vi "Obtain Request Events.vi"(8 "error in":errorcluster, 10 "Create New? (F)":bool) -> (0 "error out":errorcluster, 2 "Sequence Engine Request Events":T1)   [LabVIEW 2021, in "Sequence Engine.lvlib"]
doc: "This VI Obtains/Creates the Requests events that will be used for other modules to communicate with the module that owns this VI. These Requests events will be accessed only via Public API methods for this module.\n\n<b>NOTE</b>: The contents of this VI are automatically generated and modified by the <b>Tools > DQMH Consortium > DQMH</b> utilities. Consider using those utilities instead of making your own modifications to this VI.\n_____\nBased on DQMH Dev Tools: Project Template 7.1.1.1528."
uses:
  Sequence Engine.lvlib
  Request Events--cluster.ctl
  Stop Argument--cluster.ctl
  Show Panel Argument--cluster.ctl
  Hide Panel Argument--cluster.ctl
  Get Module Execution Status Argument--cluster.ctl
  Show Diagram Argument--cluster.ctl
  REQ Run Sequence Argument--cluster.ctl
  Request to stop testing Argument--cluster.ctl
  Init Test Context Argument--cluster.ctl
  Sequence Context.ctl
  Classes/Sequence Engine/Sequence Engine.lvclass
panel:
  # "NOTE: The contents of this VI are automatically generated and modified by the Tools > DQMH Consortium > DQMH utilities. Consider using those utilities instead of making your own modifications to this VI."
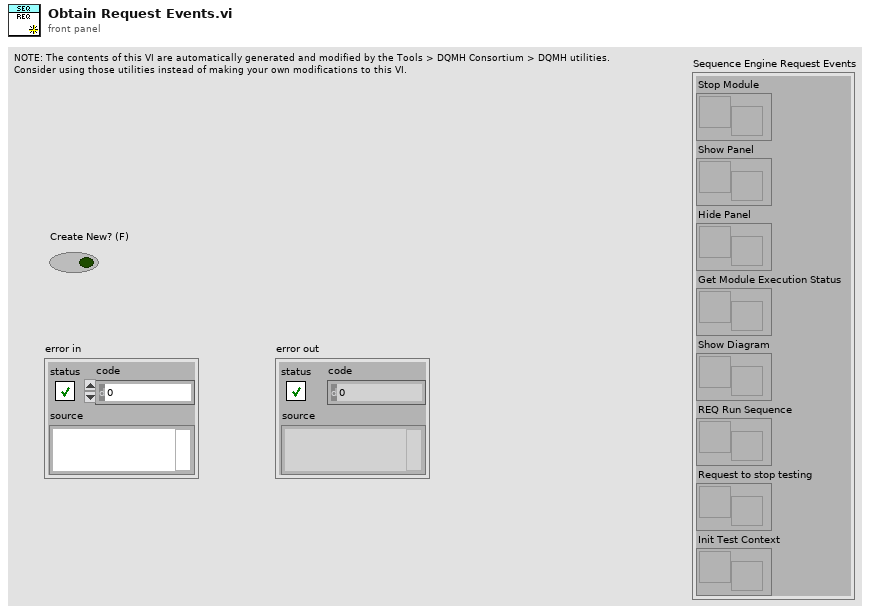
[diagram p1: front panel]
types:
  T1 = typedef "Sequence Engine.lvlib/Request Events--cluster.ctl" = cluster{"Stop Module":refnum<user-event>, "Show Panel":refnum<user-event>, "Hide Panel":refnum<user-event>, "Get Module Execution Status":refnum<user-event>, "Show Diagram":refnum<user-event>, "REQ Run Sequence":refnum<user-event>, "Request to stop testing":refnum<user-event>, "Init Test Context":refnum<user-event>}
  T2 = typedef "Sequence Engine.lvlib/Init Test Context Argument--cluster.ctl" = cluster{"Sequence Context":T3}
  T3 = typedef "Sequence Engine.lvlib/Sequence Engine.lvclass/Sequence Context.ctl" = cluster{"Execution Mode":enum16{"Production", "MSA1", "Trial"}, "Username":string, "Is Simulation":bool, "Hardware Map":string}
  T4 = typedef "Sequence Engine.lvlib/Request to stop testing Argument--cluster.ctl" = cluster{"Boolean":bool}
  T5 = typedef "Sequence Engine.lvlib/REQ Run Sequence Argument--cluster.ctl" = cluster{"Run.Start JSON":string}
  T6 = typedef "Sequence Engine.lvlib/Hide Panel Argument--cluster.ctl" = cluster{"Hide Panel?":bool}
  T7 = typedef "Sequence Engine.lvlib/Show Panel Argument--cluster.ctl" = cluster{"Show Panel?":bool}
  T8 = typedef "Sequence Engine.lvlib/Show Diagram Argument--cluster.ctl" = cluster{"Debug?":bool}
  T9 = typedef "Sequence Engine.lvlib/Get Module Execution Status Argument--cluster.ctl" = cluster{"Running?":bool}
  T10 = typedef "Sequence Engine.lvlib/Stop Argument--cluster.ctl" = cluster{"Origin":string, "Exit via Stop Module Req?":bool, "Wait for Module to stop?":bool}
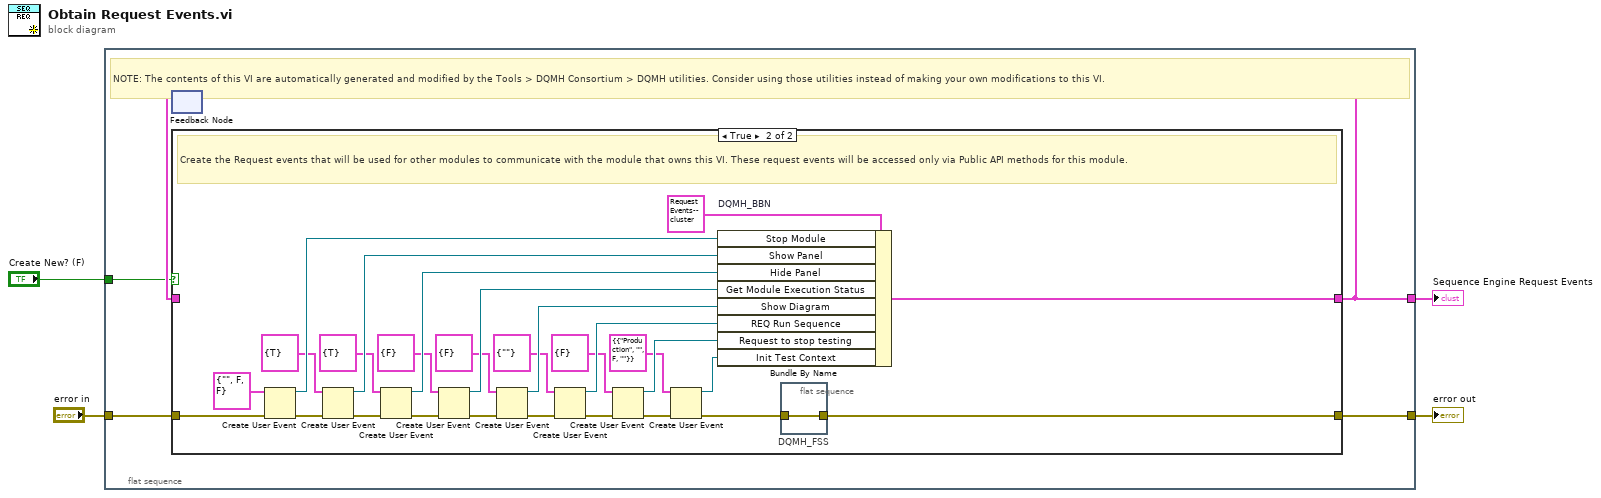
[diagram p0: block diagram]
diagram:
  n1 = flat-sequence {
    tunnel: [w9] -> w4
    tunnel: "error in" -> [w8]
    tunnel: [w6] -> w2
    tunnel: "Create New? (F)" -> [w5]
    frame #0 {
      # "NOTE: The contents of this VI are automatically generated and modified by the Tools > DQMH Consortium > DQMH utilities. Consider using those utilities instead of making your own modifications to this VI."
      n2 = feedback #1() -> (w7:T1)  [unwired: 1 in]
      n3 = case shown="True" w5 {
        tunnel: [w10 w29] -> w9
        tunnel: w8 -> [w10 w39]
        tunnel: [w11 w36] -> w6
        tunnel: w7 -> [w11 _]
        frame False {
          # "Obtain the Request events that were created in a previous call to this VI."
        }
        frame True {
          # "Create the Request events that will be used for other modules to communicate with the module that owns this VI. These request events will be accessed only via Public API methods for this module."
          n4 = Create User Event(user event datatype=T10 {"Origin"="", "Exit via Stop Module Req?"=FALSE, "Wait for Module to stop?"=FALSE} ("Stop Argument"), error in=w39) -> (user event=w37:refnum<user-event>, error out=w34:errorcluster)
          n5 = Create User Event(user event datatype=T7 {"Show Panel?"=TRUE} ("Show Panel Argument"), error in=w34) -> (user event=w33:refnum<user-event>, error out=w32:errorcluster)
          n6 = Create User Event(user event datatype=T6 {"Hide Panel?"=TRUE} ("Hide Panel Argument"), error in=w32) -> (user event=w31:refnum<user-event>, error out=w30:errorcluster)
          n7 = Create User Event(user event datatype=T9 {"Running?"=FALSE} ("Get Module Execution Status Argument"), error in=w30) -> (user event=w27:refnum<user-event>, error out=w28:errorcluster)
          n8 = Create User Event(user event datatype=T8 {"Debug?"=FALSE} ("Show Diagram Argument"), error in=w28) -> (user event=w24:refnum<user-event>, error out=w25:errorcluster)
          n9 = Create User Event(user event datatype=T5 {"Run.Start JSON"=""} ("REQ Run Sequence Argument"), error in=w25) -> (user event=w19:refnum<user-event>, error out=w20:errorcluster)
          n10 = Create User Event(user event datatype=T4 {"Boolean"=FALSE} ("Request to stop testing Argument"), error in=w20) -> (user event=w16:refnum<user-event>, error out=w17:errorcluster)
          n11 = Create User Event(user event datatype=T2 {"Sequence Context"={"Execution Mode"=enum."Production", "Username"="", "Is Simulation"=FALSE, "Hardware Map"=""}} ("Init Test Context Argument"), error in=w17) -> (user event=w13:refnum<user-event>, error out=w14:errorcluster)
          n12 = Bundle By Name "DQMH_BBN"(cluster=T1 {"Stop Module"=refnum, "Show Panel"=refnum, "Hide Panel"=refnum, "Get Module Execution Status"=refnum, "Show Diagram"=refnum, "REQ Run Sequence"=refnum, "Request to stop testing"=refnum, "Init Test Context"=refnum} ("output cluster"), "Stop Module"=w37, "Show Panel"=w33, "Hide Panel"=w31, "Get Module Execution Status"=w27, "Show Diagram"=w24, "REQ Run Sequence"=w19, "Request to stop testing"=w16, "Init Test Context"=w13) -> (w36:T1)
          n13 = flat-sequence "DQMH_FSS" {
            tunnel: w14 -> [w40]
            tunnel: [w40] -> w29
            frame #0 {
            }
          }
        }
      }
      n14 = feedback-in #1(w6) -> ()
    }
  }
  "Sequence Engine Request Events" <- w2
  "error out" <- w4
